vi "Power Max Read Single.vi"(8 "error in":errorcluster, 11 "Cycler in":refnum<class "Cycler.lvclass">) -> (0 "error out":errorcluster, 1 "Changed or First Call?":bool, 2 "Power Max SP":dbl, 3 "Cycler out":refnum<class "Cycler.lvclass">)   [LabVIEW 2023, in "Cycler.lvclass"]
uses:
  Cycler.lvclass
  Cycler.lvclass/Cycler.ctl
  Low Level Capabilities/Power/Power Limit/Power Limit.lvclass
panel:
  in  "Channel Index":i32=1
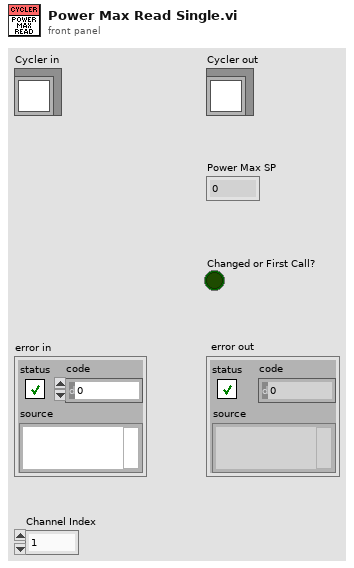
[diagram p1: front panel]
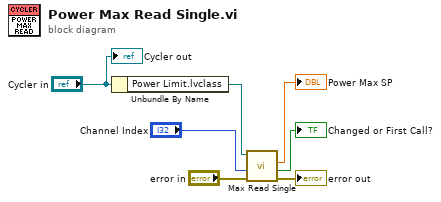
[diagram p0: block diagram]
diagram:
  n1 = Unbundle By Name("Cycler in") -> ("Power Limit.lvclass"=w7:refnum<class "Power Limit.lvclass">)
  n2 = call-dynamic "Max Read Single.vi"("error in"="error in", "Channel Index"="Channel Index", "Max Power Limit in"=w7) -> ("error out"=→"error out":errorcluster, "Changed or First Call?"=→"Changed or First Call?":bool, "Power Max SP"=→"Power Max SP":dbl)  [unwired: 5 in, 1 out]
  "Cycler out" <- "Cycler in"
